vi "Binary Search.vi"() -> ()   [LabVIEW 2009]
panel:
  out "Numeric 2":fxp<+/-,33,17> format="%.22g"
  out "Numeric":fxp<+/-,33,17> format="%.22g"
  in  "Array":fxp<+/-,32,16>[](array[numeric])=[-1.0, -1.0, -0.9656982421875, -0.932525634765625, -0.900390625, -0.869293212890625, -0.839111328125, -0.809783935546875, -0.781280517578125, -0.7535400390625, -0.726531982421875, -0.7001953125, -0.67449951171875, -0.6494140625, -0.6248779296875, -0.600860595703125, -0.577362060546875, -0.5543212890625, -0.531707763671875, -0.509521484375, -0.48773193359375, -0.46630859375, -0.445220947265625, -0.424468994140625, -0.404022216796875, -0.38385009765625, -0.363983154296875, -0.344329833984375, -0.324920654296875, -0.30572509765625, -0.2867431640625, -0.2679443359375, -0.24932861328125, -0.230865478515625, -0.212554931640625, -0.194366455078125, -0.17633056640625, -0.15838623046875, -0.140533447265625, -0.122772216796875, -0.1051025390625, -0.087493896484375, -0.069915771484375, -0.052398681640625, -0.034912109375, -0.0174560546875, 0.0, 0.0174560546875, 0.034912109375, 0.052398681640625, 0.069915771484375, 0.087493896484375, 0.1051025390625, 0.122772216796875, 0.140533447265625, 0.15838623046875, 0.17633056640625, 0.194366455078125, 0.212554931640625, 0.230865478515625, 0.24932861328125, 0.2679443359375, 0.2867431640625, 0.30572509765625, 0.324920654296875, 0.344329833984375, 0.363983154296875, 0.38385009765625, 0.404022216796875, 0.424468994140625, 0.445220947265625, 0.46630859375, 0.48773193359375, 0.509521484375, 0.531707763671875, 0.5543212890625, 0.577362060546875, 0.600860595703125, 0.6248779296875, 0.6494140625, 0.67449951171875, 0.7001953125, 0.726531982421875, 0.7535400390625, 0.781280517578125, 0.809783935546875, 0.839111328125, 0.869293212890625, 0.900390625, 0.932525634765625, 0.9656982421875]
  in  "Y":fxp<+/-,32,16>
  in  "X":fxp<+/-,32,16>
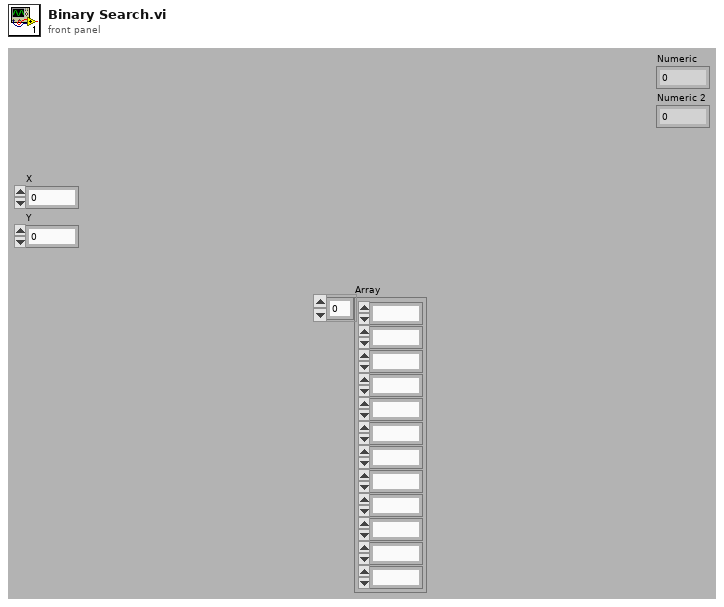
[diagram p1: front panel]
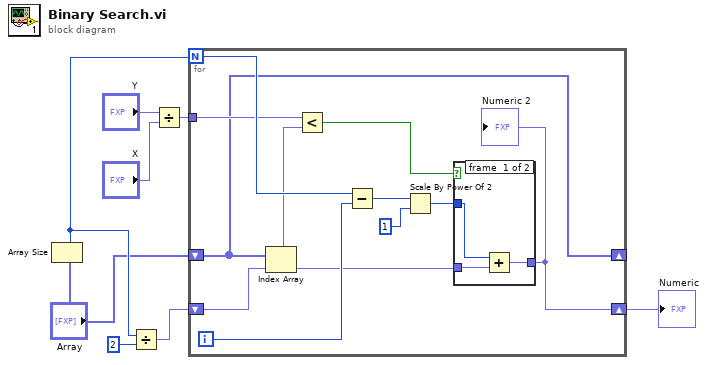
[diagram p0: block diagram]
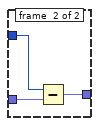
[diagram p2: hidden frame]
diagram:
  n1 = Array Size(array="Array") -> (size(s)=w5:i32)
  n2 = Divide(x=w5, y=2) -> (x/y=w3:fxp<+/-,32,16>)
  n3 = Divide(x="Y", y="X") -> (x/y=w6:fxp<+/-,64,33>)
  n4 = for {
    N: w5 -> [w15]
    tunnel: w6 -> [w11]
    shift-right: [w12] -> w1
    shift-left: w3 -> [w18]
    shift-right: [w10] -> _
    shift-left: "Array" -> [w10]
    i -> [w14]
    n5 = Index Array(array=w10, index=w18) -> (element=w9:fxp<+/-,32,16>)
    n6 = Less?(x=w11, y=w9) -> (x < y?=w19:bool)
    n7 = Subtract(x=w15, y=w14) -> (x-y=w16:i32)
    n8 = Scale By Power Of 2(n=w16, x=i16 1) -> (x*2^n=w13:i16)
    n9 = case shown="True" w19 {
      tunnel: w9 -> [w21 w24]
      tunnel: w13 -> [w20 w25]
      tunnel: [w22 w23] -> w12
      frame #0 {
        n10 = Add(x=w20, y=w21) -> (x+y=w22:fxp<+/-,33,17>)
      }
      frame #1 {
        n11 = Subtract(x=w25, y=w24) -> (x-y=w23:fxp<+/-,33,17>)
      }
    }
    "Numeric 2" <- w12
  }
  "Numeric" <- w1
